vi "REPORT_DATES_recolor_statuses.vi"(6 "Recolor? (T)":bool=TRUE, 8 "error_in":errorcluster, 10 "record_statuses":T1[](array[typedef]), 11 "listbox_ref":refnum<vi>) -> (0 "error_out":errorcluster)   [LabVIEW 2019]
uses:
  typedef/REPORT_DATES_statuses.ctl
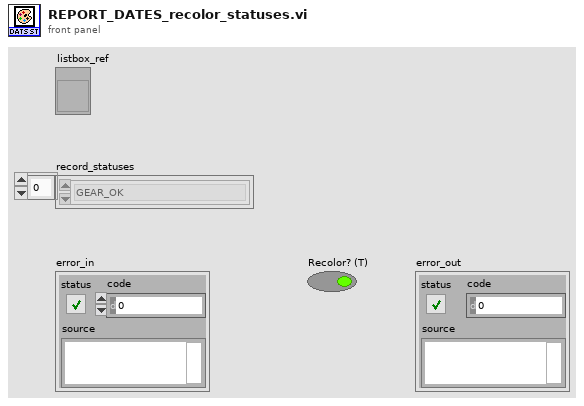
[diagram p1: front panel]
types:
  T1 = typedef "REPORT_DATES_statuses.ctl" = enum16{"GEAR_OK", "GEAR_NOK", "GEAR_interrupted", "GEAR_in_operation", "GEAR_unexpected"}
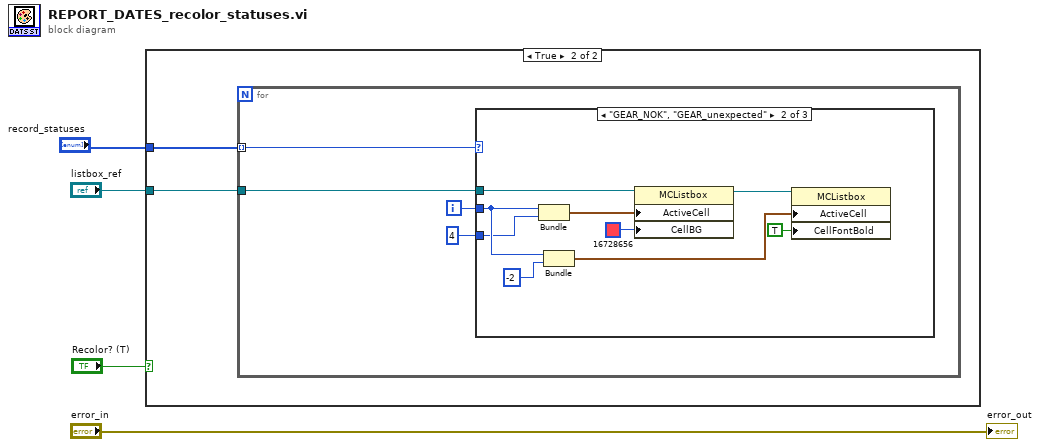
[diagram p0: block diagram]
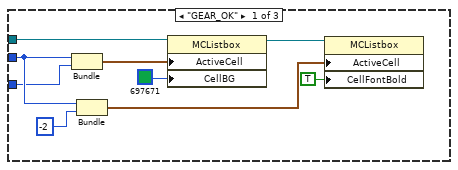
[diagram p3: hidden frame]
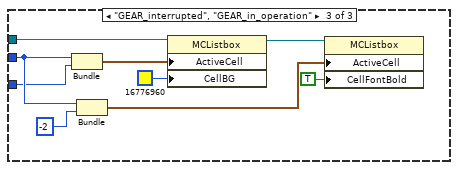
[diagram p4: hidden frame]
diagram:
  n1 = case shown="True" "Recolor? (T)" {
    tunnel: "record_statuses" -> [_ w5]
    tunnel: "listbox_ref" -> [_ w6]
    frame False {
    }
    frame True {
      n2 = for {
        tunnel: w6 -> [w10]
        tunnel: w5 -> [w9] mode=indexing
        i -> [w8]
        n3 = case shown="\"GEAR_NOK\", \"GEAR_unexpected\"" w9 {
          tunnel: w10 -> [w18 w27 w36]
          tunnel: w8 -> [w17 w26 w35]
          tunnel: 4 -> [w11 w20 w29]
          frame "GEAR_OK" {
            n4 = Bundle(w17, w11) -> (w19:cluster{i32, i32})  [unwired: 1 in]
            n5 = Bundle(w17, -2) -> (w14:cluster{i32, i32})  [unwired: 1 in]
            n6 = property on="Property Node" class="MCListbox"(reference=w18, "ActiveCell"=w19, "CellBG"=u32 697671) -> (reference out=w15:refnum<vi>)  [unwired: 1 in, 1 out]
            n7 = property on="Property Node" class="MCListbox"(reference=w15, "ActiveCell"=w14, "CellFontBold"=TRUE ("Active Cell:Cell Font:Bold")) -> ()  [unwired: 1 in, 2 out]
          }
          frame "GEAR_NOK", "GEAR_unexpected" {
            n8 = Bundle(w26, w20) -> (w28:cluster{i32, i32})  [unwired: 1 in]
            n9 = Bundle(w26, -2) -> (w23:cluster{i32, i32})  [unwired: 1 in]
            n10 = property on="Property Node" class="MCListbox"(reference=w27, "ActiveCell"=w28, "CellBG"=u32 16728656) -> (reference out=w24:refnum<vi>)  [unwired: 1 in, 1 out]
            n11 = property on="Property Node" class="MCListbox"(reference=w24, "ActiveCell"=w23, "CellFontBold"=TRUE ("Active Cell:Cell Font:Bold")) -> ()  [unwired: 1 in, 2 out]
          }
          frame "GEAR_interrupted", "GEAR_in_operation" {
            n12 = Bundle(w35, w29) -> (w37:cluster{i32, i32})  [unwired: 1 in]
            n13 = Bundle(w35, -2) -> (w32:cluster{i32, i32})  [unwired: 1 in]
            n14 = property on="Property Node" class="MCListbox"(reference=w36, "ActiveCell"=w37, "CellBG"=u32 16776960) -> (reference out=w33:refnum<vi>)  [unwired: 1 in, 1 out]
            n15 = property on="Property Node" class="MCListbox"(reference=w33, "ActiveCell"=w32, "CellFontBold"=TRUE ("Active Cell:Cell Font:Bold")) -> ()  [unwired: 1 in, 2 out]
          }
        }
      }
    }
  }
  "error_out" <- "error_in"
